vi "Set Coils.vi"(10 "Coils":refnum<vi>, 11 "DAM0404D in":refnum<class "DAM0404D.lvclass">) -> (3 "DAM0404D out":refnum<class "DAM0404D.lvclass">)   [LabVIEW 2016, in "DAM0404D.lvlib" / "DAM0404D.lvclass"]
uses:
  DAM0404D.lvclass
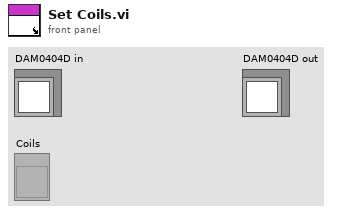
[diagram p1: front panel]
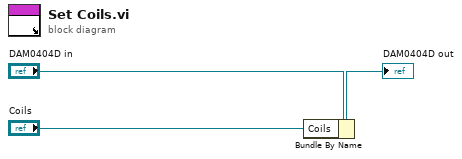
[diagram p0: block diagram]
diagram:
  n1 = Bundle By Name(cluster="DAM0404D in", "Coils"="Coils") -> (→"DAM0404D out":refnum<class "DAM0404D.lvclass">)
